vi "Generate Digital Pulse (mSec).vi"(9 "invert pulse (F)":bool, 10 "pulse width (mSec)":u32, 11 "FPGA digital output":refnum<k21>="Port0/DIO0") -> ()   [LabVIEW 2017, in "NI_Robotics_FPGA Utilities.lvlib"]
uses:
  <vilib>/robotics/Utilities/FPGA Utilities/NI_Robotics_FPGA Utilities.lvlib
  <vilib>/eio/EIONode/EIONode.xnode
  <vilib>/rvi/eio/common/nirviEmuTemplateMethod_errors.vi
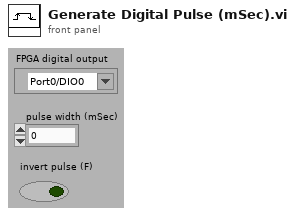
[diagram p1: front panel]
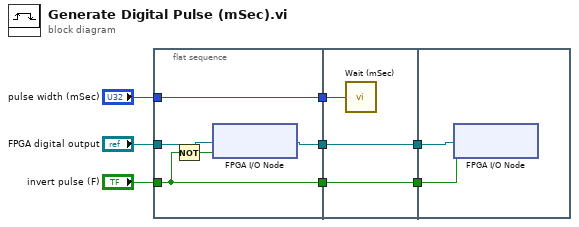
[diagram p0: block diagram]
diagram:
  n1 = flat-sequence {
    tunnel: "FPGA digital output" -> [w13]
    tunnel: [w12] -> w8
    tunnel: "pulse width (mSec)" -> [w11]
    tunnel: [w11] -> w7
    tunnel: "invert pulse (F)" -> [w10]
    tunnel: [w10] -> w2
    tunnel: w8 -> [w16]
    tunnel: w7 -> [w15]
    tunnel: [w16] -> w6
    tunnel: w2 -> [w14]
    tunnel: [w14] -> w1
    tunnel: w6 -> [w18]
    tunnel: w1 -> [w17]
    frame #0 {
      n2 = Not(x=w10) -> (.not. x?=w9:bool)
      n3 = xnode "FPGA I/O Node"("I/O Item"=w9, "FPGA I/O In"=w13) -> ("FPGA I/O Out"=w12:refnum<k21>)
    }
    frame #1 {
      n4 = call "Wait (mSec)"("Count(mSec)"=w15) -> ()  [unwired: 1 out]
    }
    frame #2 {
      n5 = xnode "FPGA I/O Node"("I/O Item"=w17, "FPGA I/O In"=w18) -> ()  [unwired: 1 out]
    }
  }
